vi "resultsColumnsDateDetails.vi"(10 "chValuesIn":string[](array[string]), 11 "chNamesIn":string[](array[string])) -> (2 "chValuesOut":string[](array[string]), 3 "chNamesOut":string[](array[string]))   [LabVIEW 2022 SP3]
uses:
  Globals/Meas_global.vi
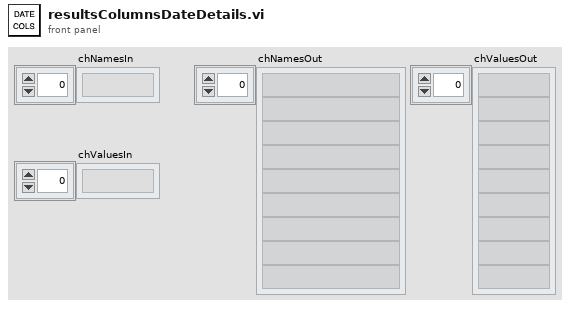
[diagram p1: front panel]
types:
  T1 = typedef "Post_Process.ctl" = enum16{"Take New Data", "Post Process Raw Data File"}
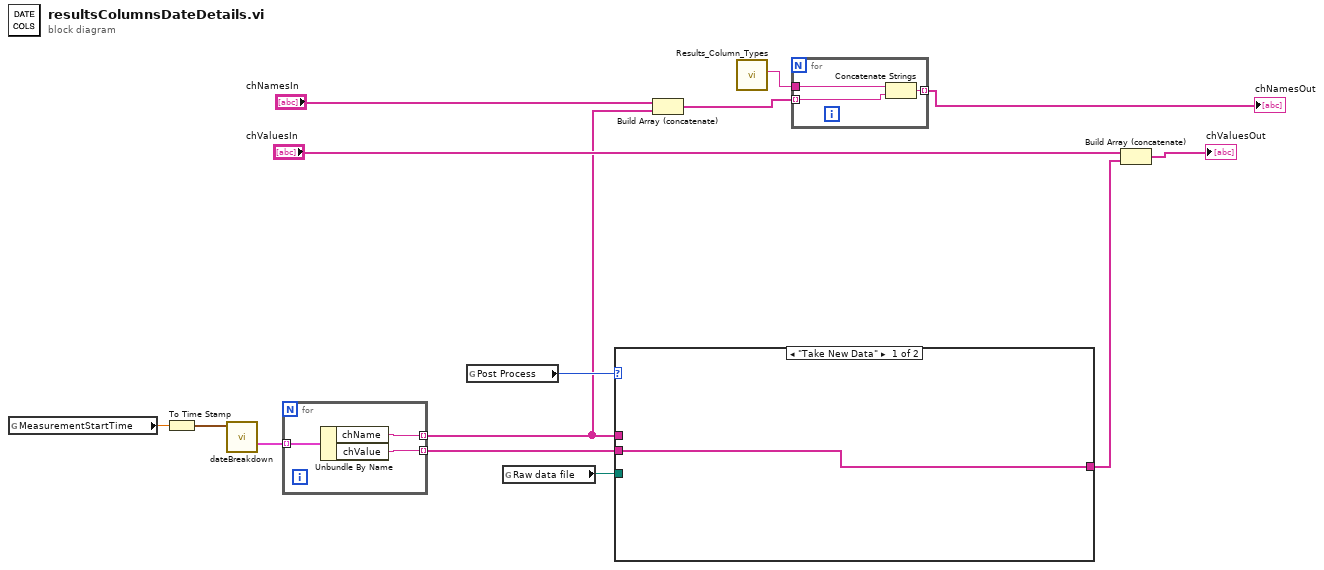
[diagram p0: block diagram]
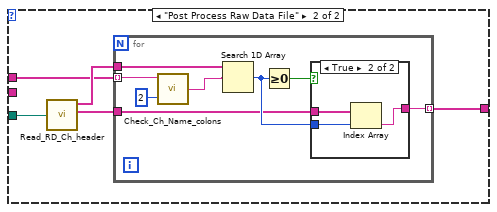
[diagram p2: hidden frame]
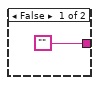
[diagram p3: hidden frame]
diagram:
  n1 = global read "Meas_global.vi" "MeasurementStartTime"() -> (w5:dbl)
  n2 = To Time Stamp(1:w5) -> (0:w4:timestamp)
  n3 = call "dateBreakdown.vi"("seconds since 1Jan1904"=w4) -> ("dateElementsArray"=w8:cluster{"chName":string, "chValue":string}[])  [unwired: 10 in]
  n4 = for {
    tunnel: w8 -> [w17] mode=indexing
    tunnel: [w16] -> w7 mode=indexing
    tunnel: [w15] -> w6 mode=indexing
    n5 = Unbundle By Name(w17) -> ("chName"=w16:string, "chValue"=w15:string)
  }
  n6 = global read "Meas_global.vi" "Post Process"() -> (w11:T1)
  n7 = global read "Meas_global.vi" "Raw data file"() -> (w10:path)
  n8 = case shown="\"Take New Data\"" w11 {
    tunnel: [w18 w19] -> w9
    tunnel: w10 -> [_ w23]
    tunnel: w7 -> [_ w20]
    tunnel: w6 -> [w18 _]
    frame "Take New Data" {
    }
    frame "Post Process Raw Data File" {
      n9 = call "Read_RD_Ch_header.vi"("Raw data file"=w23) -> ("Ch Name Out"=w22:string[], "Ch Values"=w21:string[])  [unwired: 2 out]
      n10 = for {
        tunnel: w22 -> [w31]
        tunnel: w21 -> [w28]
        tunnel: [w27] -> w19 mode=indexing
        tunnel: w20 -> [w26] mode=indexing
        n11 = call "Check_Ch_Name_colons.vi"("No of Colons"=2, "Ch Name in"=w26) -> ("Ch Name out"=w25:string)
        n12 = Search 1D Array(1D array=w31, element=w25) -> (index of element=w29:i32)  [unwired: 1 out]
        n13 = Greater Or Equal To 0?(x=w29) -> (x >= 0?=w30:bool)
        n14 = case shown="True" w30 {
          tunnel: w29 -> [_ w35]
          tunnel: w28 -> [_ w34]
          tunnel: ["" w33] -> w27
          frame False {
          }
          frame True {
            n15 = Index Array(array=w34, index=w35) -> (element=w33:string)
          }
        }
      }
    }
  }
  n16 = Build Array (concatenate)("chNamesIn", w7) -> (w3:string[])
  n17 = call "Results_Column_Types.vi"() -> ("Metadata"=w1:string)  [unwired: 9 in, 2 out]
  n18 = for {
    tunnel: w3 -> [w38] mode=indexing
    tunnel: [w37] -> w2 mode=indexing
    tunnel: w1 -> [w36]
    n19 = Concatenate Strings(w36, w38) -> (w37:string)
  }
  "chNamesOut" <- w2
  n20 = Build Array (concatenate)("chValuesIn", w9) -> (→"chValuesOut":string[])
